vi "WPI_GyroClose.vi"(8 "error in (no error)":errorcluster, 11 "GyroDevRef":T1) -> (0 "error out":errorcluster)   [LabVIEW 2013]
doc: "Closes the reference to the gyroscope you specify. Use this VI to close each gyroscope reference that you open with the Open VI.\n\nThis software is licensed. Open the labview\\readme\\WPI Robotics Library Open Source License.txt file for more information."
uses:
  <vilib>/Rock Robotics/WPI/Gyro/WPI_GyroDevRef.ctl
  <vilib>/Rock Robotics/SystemInterfaces/Typedef/FPGA_TypedefAnalogModule.ctl
  <vilib>/Rock Robotics/SystemInterfaces/AI/FPGA_AIChannel.ctl
  <vilib>/Rock Robotics/SystemInterfaces/AI/FPGA_AIGyroChannel.ctl
  <instrlib>/Sparkfun Atomic IMU/HAIOL/Sparkfun Atomic IMU.lvclass
  <instrlib>/Honeywell Compass HMC6343/HAIOL/Honeywell Compass HMC6343.lvclass
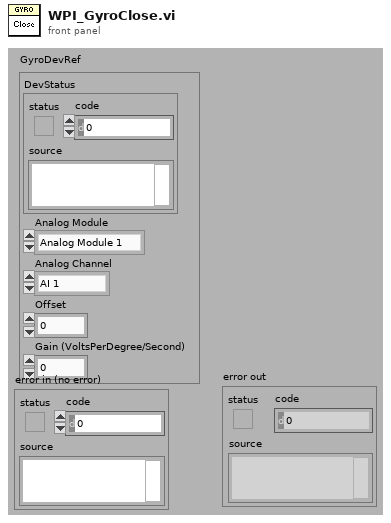
[diagram p1: front panel]
types:
  T1 = typedef "WPI_GyroDevRef.ctl" = cluster{"DevStatus":errorcluster, "Analog Module":T2, "Analog Channel":T3, "Offset":dbl, "Gain (VoltsPerDegree/Second)":dbl}
  T2 = typedef "FPGA_TypedefAnalogModule.ctl" = enum16{"Analog Module 1", "Analog Module 2"}
  T3 = typedef "FPGA_AIChannel.ctl" = enum8{"AI 1", "AI 2", "AI 3", "AI 4", "AI 5", "AI 6", "AI 7", "AI 8", "Invalid"}
  T4 = typedef "WPI_AnalogChannelDevRef.ctl" = cluster{"DevStatus":errorcluster, "Analog Module":T2, "Analog Channel":T3}
  T5 = typedef "FPGA_AIGyroChannel.ctl" = enum8{"AI 1", "AI 2", "Invalid"}
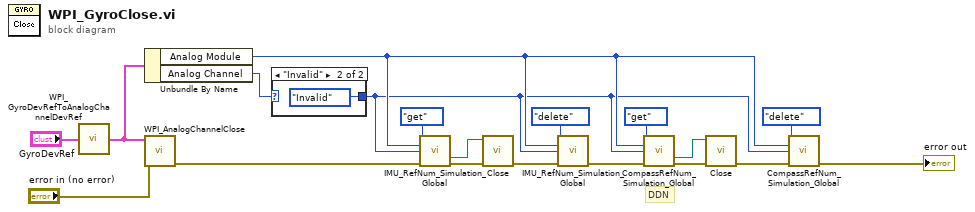
[diagram p0: block diagram]
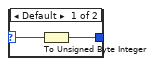
[diagram p2: hidden frame]
diagram:
  # "DDN"
  n1 = call "WPI_GyroDevRefToAnalogChannelDevRef.vi"("GyroDeviceRef"="GyroDevRef") -> ("AIDeviceRef"=w15:T4)  [unwired: 4 out]
  n2 = Unbundle By Name(w15) -> ("Analog Module"=w4:T2, "Analog Channel"=w14:T3)
  n3 = call <vilib>:"WPI_AnalogChannelClose.vi"("error in (no error)"="error in (no error)", "AIDeviceRef"=w15) -> ("error out"=w13:errorcluster)  [unwired: 9 out]
  n4 = case shown="\"Invalid\"" w14 {
    selector: w14 -> [w21 _]
    tunnel: [w20 FPGA_AIGyroChannel."Invalid" ("Analog Channel")] -> w3
    frame Default {
      n5 = To Unsigned Byte Integer(number=w21) -> (unsigned 8bit integer=w20:u8)
    }
    frame "Invalid" {
    }
  }
  n6 = call <vilib>:"IMU_RefNum_Simulation_Global.vi"("menu"=enum16{"set", "get", "delete"}."get", "Analog Module (Module 1)"=w4, "Analog Channel"=w3, "error in (no error)"=w13) -> ("Sparkfun Atomic IMU Get"=w11:refnum<class "Sparkfun Atomic IMU.lvclass">, "error out"=w12:errorcluster)  [unwired: 10 in]
  n7 = call-dynamic "Close.vi"("error in (no error)"=w12, "Sparkfun Atomic IMU in"=w11) -> ("error out"=w9:errorcluster)  [unwired: 9 in]
  n8 = call <vilib>:"IMU_RefNum_Simulation_Global.vi"("menu"=enum16{"set", "get", "delete"}."delete", "Analog Module (Module 1)"=w4, "Analog Channel"=w3, "error in (no error)"=w9) -> ("error out"=w8:errorcluster)  [unwired: 10 in, 1 out]
  n9 = call <vilib>:"CompassRefNum_Simulation_Global.vi"("menu"=enum16{"set", "get", "delete"}."get", "Analog Module (Module 1)"=w4, "Analog Channel"=w3, "error in (no error)"=w8) -> ("Honeywell Compass HMC6343 Get"=w6:refnum<class "Honeywell Compass HMC6343.lvclass">, "error out"=w7:errorcluster)  [unwired: 10 in]
  n10 = call-dynamic "Close.vi"("error in (no error)"=w7, "Honeywell Compass HMC6343"=w6) -> ("error out"=w2:errorcluster)  [unwired: 9 in]
  n11 = call <vilib>:"CompassRefNum_Simulation_Global.vi"("menu"=enum16{"set", "get", "delete"}."delete", "Analog Module (Module 1)"=w4, "Analog Channel"=w3, "error in (no error)"=w2) -> ("error out"=→"error out":errorcluster)  [unwired: 10 in, 1 out]
